vi "PrepareChannels_2Analog.vi"(0 "Real stim channel":tag="pciDAQ/ao0", 1 "Sampling Rate (Hz)":dbl=100000.0, 2 "Onboard counter":tag="pciDAQ/ctr0", 5 "Sham stim channel":tag="pciDAQ/ao2", 7 "OEP sample clock in":tag="/pciDAQ/PFI0", 9 "Num Pulses":u32=1 min=1, 11 "error in":errorcluster, 12 "Pulse Type":enum16{"Monophasic", "Biphasic"}(ring)=enum."Biphasic", 13 "Pulse Width (ms)":dbl=0.09) -> (3 "Waveform Graph":waveform(dbl)(graph), 4 "Real stim task":refnum<k21>, 6 "Sham stim task":refnum<k21>, 10 "ctr task out":refnum<k21>, 15 "Error out":errorcluster)   [LabVIEW 2017]
uses:
  <vilib>/DAQmx/configure/timing.llb/DAQmx Timing (Use Waveform).vi
  <vilib>/DAQmx/create/channels.llb/DAQmx Create Channel (AO-Voltage-Basic).vi
  <vilib>/DAQmx/create/channels.llb/DAQmx Create Channel (CI-Count Edges).vi
  <resource>/objmgr/daqmx.rc
panel:
  in  "Amplitude (Volts)":dbl=1.0
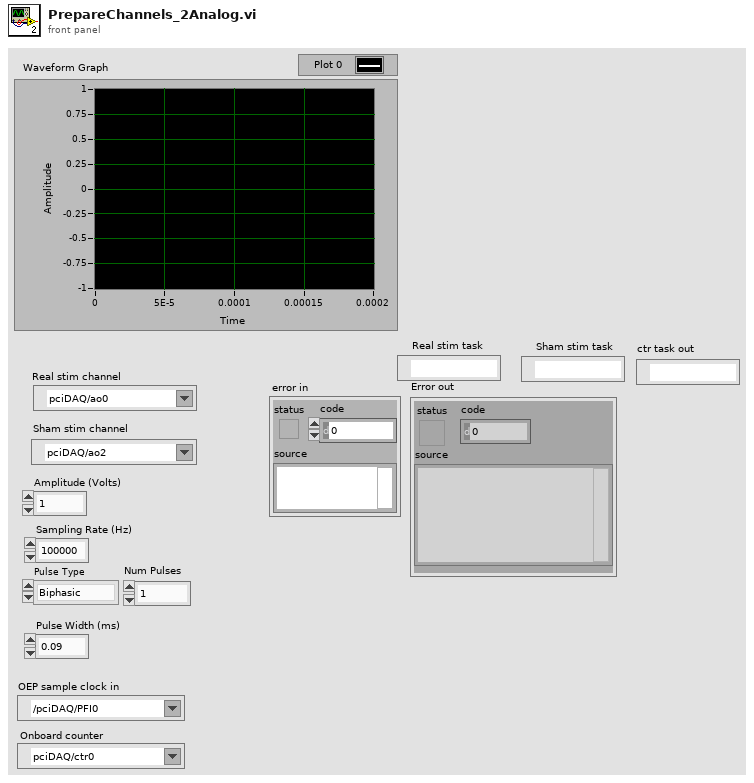
[diagram p1: front panel]
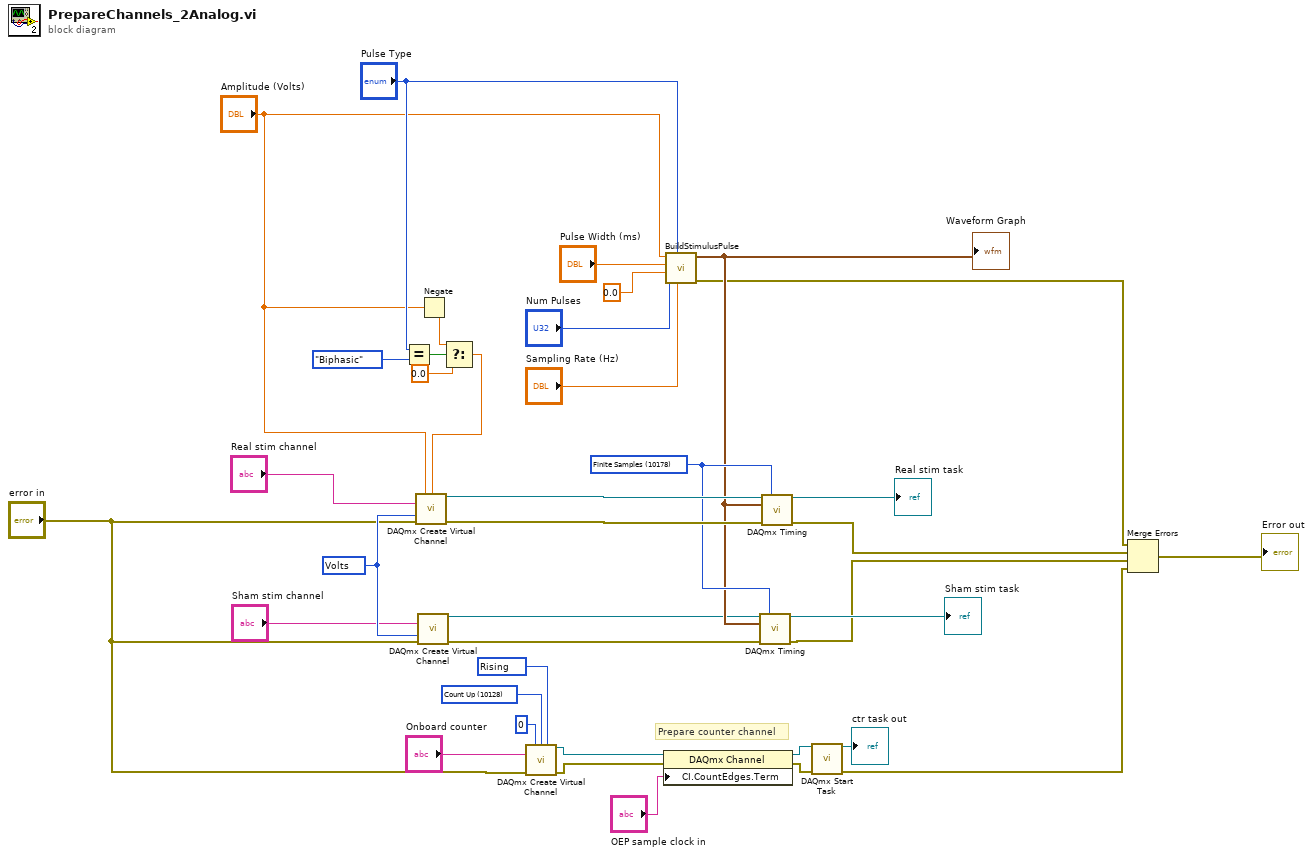
[diagram p0: block diagram]
diagram:
  w13 = 10178 items=["Finite Samples"=10178, "Continuous Samples"=10123, "Hardware Timed Single Point"=12522] ("sample mode")
  w20 = 10280 items=["Rising"=10280, "Falling"=10171] ("edge")
  w21 = 10128 items=["Count Up"=10128, "Count Down"=10124, "Externally Controlled"=10326] ("count direction")
  w12 = 10348 items=["Volts"=10348, "From Custom Scale"=10065] ("units")
  # "Prepare counter channel"
  n1 = Equal?(x="Pulse Type", y=enum16{"Monophasic", "Biphasic"}."Biphasic") -> (x = y?=w30:bool)
  n2 = call-poly <vilib>:"DAQmx Create Virtual Channel.vi"("physical channels"="Sham stim channel", "units"=w12, "error in"="error in") -> ("task out"=w10:refnum<k21>, "error out"=w9:errorcluster)  [unwired: 11 in]
  n3 = Negate(x="Amplitude (Volts)") -> (-x=w28:dbl)
  n4 = Select(t=w28, s=w30, f=0.0) -> (s? t:f=w26:dbl)
  n5 = call-poly <vilib>:"DAQmx Create Virtual Channel.vi"("maximum value"="Amplitude (Volts)", "minimum value"=w26, "physical channels"="Real stim channel", "units"=w12, "error in"="error in") -> ("task out"=w34:refnum<k21>, "error out"=w33:errorcluster)  [unwired: 9 in]
  n6 = call-poly <vilib>:"DAQmx Create Virtual Channel.vi"("initial count"=u32 0, "count direction"=w21, "edge"=w20, "counter"="Onboard counter", "error in"="error in") -> ("task out"=w23:refnum<k21>, "error out"=w22:errorcluster)  [unwired: 9 in]
  n7 = property class="DAQmx Channel"(reference=w23, error in=w22, "CI.CountEdges.Term"="OEP sample clock in") -> (reference out=w19:refnum<k21>, error out=w18:errorcluster)
  n8 = call "BuildStimulusPulse.vi"("Sampling Rate (Hz)"="Sampling Rate (Hz)", "Pulse Type"="Pulse Type", "Num Pulses"="Num Pulses", "Inter-Pulse Interval (ms)"=0.0, "Pulse Width (ms)"="Pulse Width (ms)", "Amplitude (Volts)"="Amplitude (Volts)") -> ("error out"=w2:errorcluster, "Waveform Out"=w11:waveform(dbl))  [unwired: 3 in, 1 out]
  "Waveform Graph" <- w11
  n9 = call-poly <vilib>:"DAQmx Timing.vi"("task/channels in"=w10, "sample mode"=w13, "waveform"=w11, "error in"=w9) -> ("task out"=→"Sham stim task":refnum<k21>, "error out"=w4:errorcluster)  [unwired: 10 in]
  n10 = call-poly <vilib>:"DAQmx Timing.vi"("task/channels in"=w34, "sample mode"=w13, "waveform"=w11, "error in"=w33) -> ("task out"=→"Real stim task":refnum<k21>, "error out"=w6:errorcluster)  [unwired: 10 in]
  n11 = call <vilib>:"DAQmx Start Task.vi"("task/channels in"=w19, "error in"=w18) -> ("task out"=→"ctr task out":refnum<k21>, "error out"=w3:errorcluster)  [unwired: 12 in]
  n12 = Merge Errors(w2, w6, w4, w3) -> (→"Error out":errorcluster)
